vi "MainGUI.vi"() -> ()   [LabVIEW 2017, in "MainGUI.lvlib"]
uses:
  MainGUI.lvlib
  Communication/SubVIs/QueueRepo.Action.ctl
  <vilib>/Utility/miscctls.llb/LVPositionTypeDef.ctl
  GUIReferences.Action.ctl
  Communication/Communication.lvlib
panel:
  in  "Exit App":bool
  in  "Buttons":enum32{"Standard Button", "Standard Button 2"}(radio)
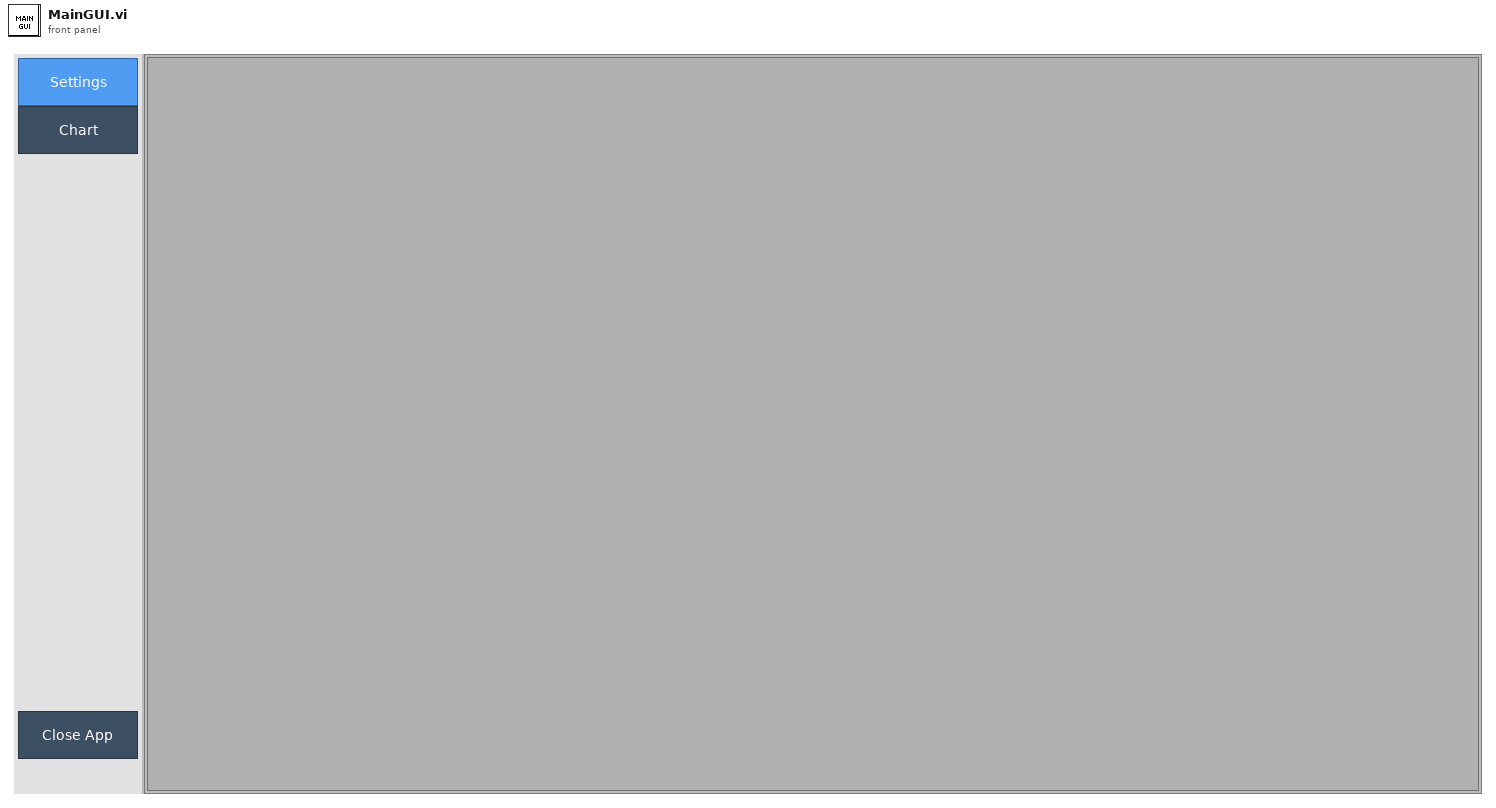
[diagram p1: front panel]
types:
  T1 = typedef "Communication.lvlib/QueueRepo.Action.ctl" = enum16{"Add", "Get", "Destroy", "Get All", "Clear"}
  T2 = typedef "MainGUI.lvlib/GUIReferences.Action.ctl" = enum16{"Get", "Register", "Unregister"}
  T3 = typedef "LVPositionTypeDef.ctl" = cluster{"Left":i32, "Top":i32}
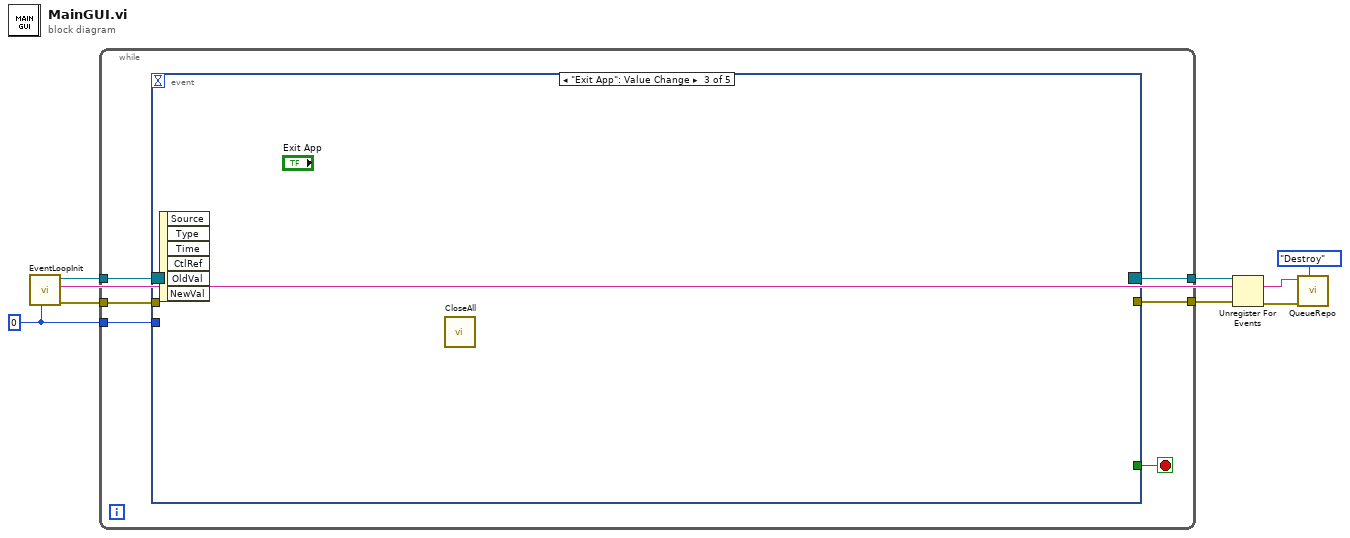
[diagram p0: block diagram]
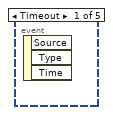
[diagram p2: hidden frame]
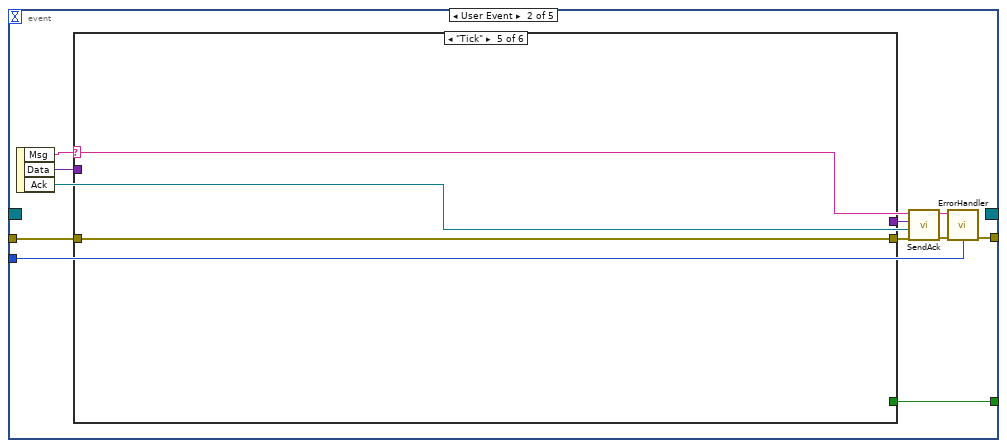
[diagram p3: hidden frame]
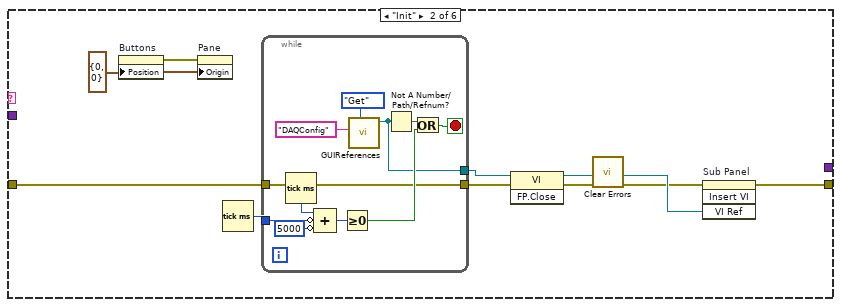
[diagram p5: hidden frame]
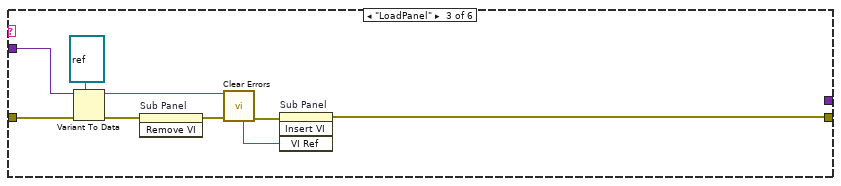
[diagram p6: hidden frame]
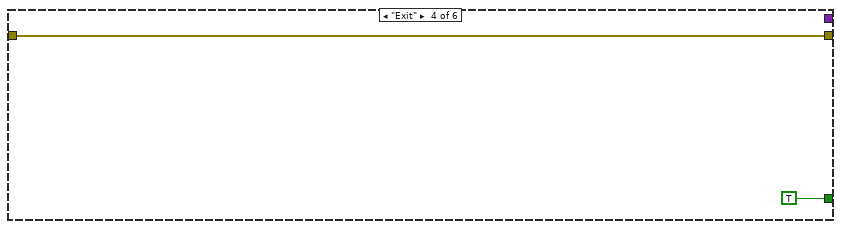
[diagram p7: hidden frame]
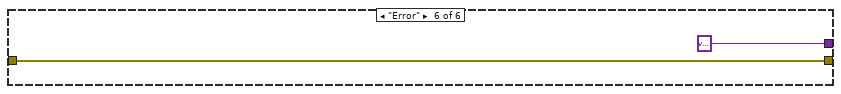
[diagram p8: hidden frame]
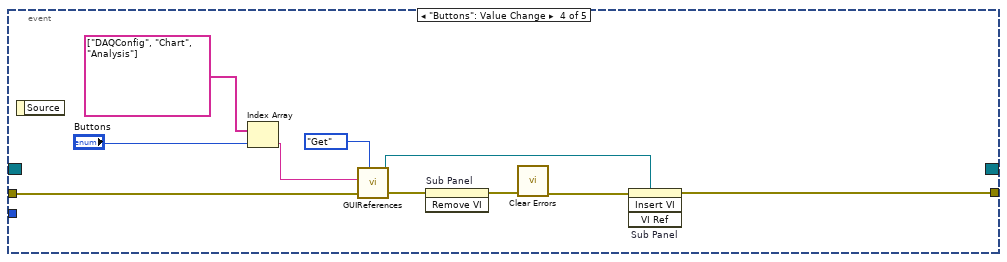
[diagram p9: hidden frame]
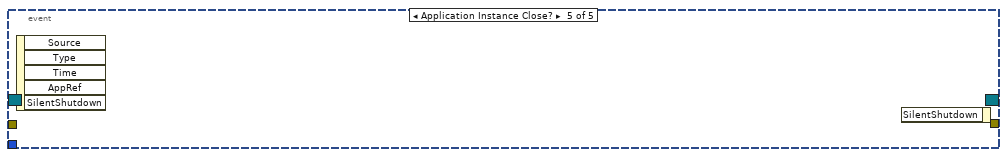
[diagram p10: hidden frame]
diagram:
  w6 = 0 ("Instance")
  n1 = call "EventLoopInit.vi"("Instance"=w6) -> ("error out"=w7:errorcluster, "Loop Name"=w3:string, "Event Registration Refnum"=w8:refnum<event-registration>)  [unwired: 8 in]
  n2 = while {
    tunnel: w8 -> [w14]
    tunnel: w7 -> [w13]
    tunnel: w6 -> [w12]
    tunnel: [w10] -> w5
    tunnel: [w9] -> w4
    stop <- w11 stop-if-true
    n3 = event shown="[2] \"Exit App\": Value Change" {
      selector: w14 -> [_ _ _ _ _]
      dyn-events: [_ _ _ _ _] -> w10
      timeout: _ -> [_ _ _ _ _]
      tunnel: w13 -> [_ w23 _ w62 _]
      tunnel: [_ w19 _ w66 _] -> w9
      tunnel: w12 -> [_ w18 _ _ _]
      tunnel: [_ w15 _ _ _] -> w11
      event Timeout {
        n4 = event-data() -> ()  [unwired: 1 in, 3 out]
      }
      event User Event {
        n5 = event-data() -> ("Msg"=w20:string, "Data"=w24:variant, "Ack"=w22:refnum<notifier>)  [unwired: 1 in]
        n6 = case shown="\"Tick\"" w20 {
          tunnel: w24 -> [_ _ w52 _ _ _]
          tunnel: w23 -> [w25 w32 w54 w56 w57 w58]
          tunnel: [_ _ _ _ _ variant] -> w17
          tunnel: [w25 w31 w47 w56 w57 w58] -> w16
          tunnel: [_ _ _ TRUE _ _] -> w15
          frame Default {
          }
          frame "Init" {
            w34 = T3 {"Left"=0, "Top"=0} ("Position")
            n7 = property on="Buttons" class="RadioBtnsControl (strict)"("Position"=w34) -> (error out=w35:errorcluster)  [unwired: 2 in, 1 out]
            n8 = property on="Pane" class="Pane"(error in=w35, "Origin"=w34) -> ()  [unwired: 1 in, 2 out]
            n9 = Tick Count (ms)() -> (millisecond timer value=w33:u32)
            n10 = while {
              tunnel: w33 -> [w43]
              tunnel: w32 -> [w36]
              tunnel: [w37] -> w30
              tunnel: [w36] -> w29
              stop <- w40 stop-if-true
              n11 = Tick Count (ms)() -> (millisecond timer value=w44:u32)
              n12 = Compound Arithmetic op=ADD(w44, invert w43, invert u32 5000 ("value")) -> (w41:u32)
              n13 = Greater Or Equal To 0?(x=w41) -> (x >= 0?=w38:bool)
              n14 = call "GUIReferences.vi"("Action"=GUIReferences.Action."Get", "String"="DAQConfig") -> ("VI Refnum"=w37:refnum<vi>)  [unwired: 8 in, 1 out]
              n15 = Not A Number/Path/Refnum?(number/path/refnum=w37) -> (NaN/Path/Refnum?=w39:bool)
              n16 = Or(x=w39, y=w38) -> (x .or. y?=w40:bool)
            }
            n17 = invoke class="VI" method="FP.Close"(reference=w30, error in=w29) -> (reference out=w28:refnum<vi>, error out=w27:errorcluster)  [unwired: 1 in, 1 out]
            n18 = call <vilib>:"Clear Errors.vi"("error in (no error)"=w27) -> ("error out"=w26:errorcluster)  [unwired: 5 in, 1 out]
            n19 = invoke on="Sub Panel" class="SubPanel" method="Insert VI"(error in=w26, "VI Ref"=w28) -> (error out=w31:errorcluster)  [unwired: 2 in, 3 out]
          }
          frame "LoadPanel" {
            n20 = Variant To Data(error in=w54, type=refnum<vi> refnum ("This VI"), Variant=w52) -> (data=w50:refnum<vi>, error out=w51:errorcluster)
            n21 = invoke on="Sub Panel" class="SubPnl" method="Remove VI"(error in=w51) -> (error out=w49:errorcluster)  [unwired: 2 in, 2 out]
            n22 = call <vilib>:"Clear Errors.vi"("error in (no error)"=w49) -> ("error out"=w48:errorcluster)  [unwired: 5 in, 1 out]
            n23 = invoke on="Sub Panel" class="SubPnl" method="Insert VI"(error in=w48, "VI Ref"=w50) -> (error out=w47:errorcluster)  [unwired: 2 in, 3 out]
          }
          frame "Exit" {
          }
          frame "Tick" {
          }
          frame "Error" {
          }
        }
        n24 = call "SendAck.vi"("error in (no error)"=w16, "Ack"=w22, "Variant"=w17) -> ("error out"=w21:errorcluster)  [unwired: 8 in]
        n25 = call "ErrorHandler.vi"("Instance"=w18, "error in (no error)"=w21, "Msg"=w20) -> ("error out"=w19:errorcluster)  [unwired: 8 in]
      }
      event "Exit App": Value Change {
        n26 = event-data() -> ()  [unwired: 1 in, 6 out]
        n27 = call "CloseAll.vi"() -> ()  [unwired: 12 in]
      }
      event "Buttons": Value Change {
        n28 = event-data() -> ()  [unwired: 1 in, 1 out]
        n29 = Index Array(array=string[] ["DAQConfig", "Chart", "Analysis"], index="Buttons") -> (element=w63:string)
        n30 = call "GUIReferences.vi"("Action"=GUIReferences.Action."Get", "error in (no error)"=w62, "String"=w63) -> ("error out"=w67:errorcluster, "VI Refnum"=w69:refnum<vi>)  [unwired: 7 in]
        n31 = invoke on="Sub Panel" class="SubPnl" method="Remove VI"(error in=w67) -> (error out=w61:errorcluster)  [unwired: 2 in, 2 out]
        n32 = call <vilib>:"Clear Errors.vi"("error in (no error)"=w61) -> ("error out"=w60:errorcluster)  [unwired: 5 in, 1 out]
        n33 = invoke on="Sub Panel" class="SubPnl" method="Insert VI"(error in=w60, "VI Ref"=w69) -> (error out=w66:errorcluster)  [unwired: 2 in, 3 out]
      }
      event Application Instance Close? {
        n34 = event-data() -> ()  [unwired: 1 in, 5 out]
        n35 = event-data() -> ()  [unwired: 2 in, 1 out]
      }
    }
  }
  n36 = Unregister For Events(event registration refnum=w5, error in=w4) -> (error out=w2:errorcluster)
  n37 = call "QueueRepo.vi"("Action"=QueueRepo.Action."Destroy", "error in (no error)"=w2, "Name"=w3) -> ()  [unwired: 5 in, 4 out]
